vi "readAI.vi"(8 "error in (no error)":errorcluster, 10 "Samples To Read":i32=1000, 11 "DAQ Channel To Read":refnum<k21>) -> (0 "error out":errorcluster, 2 "Average":dbl, 3 "Samples":dbl[](array[numeric]) format="%0.2f")   [LabVIEW 2015]
uses:
  <vilib>/DAQmx/read.llb/DAQmx Read (Analog 1D DBL 1Chan NSamp).vi
  <vilib>/DAQmx/configure/timing.llb/DAQmx Timing (Sample Clock).vi
  <vilib>/DAQmx/miscellaneous.llb/DAQmx Fill In Error Info.vi
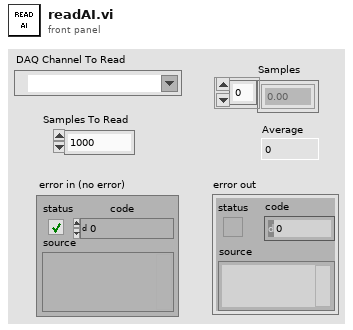
[diagram p1: front panel]
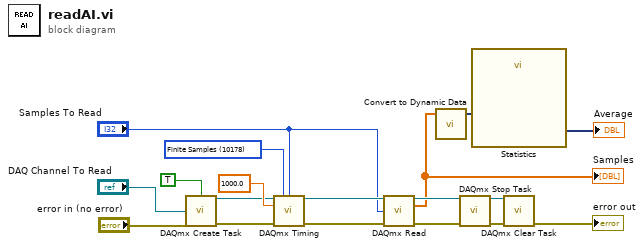
[diagram p0: block diagram]
diagram:
  w14 = 10178 items=["Finite Samples"=10178, "Continuous Samples"=10123, "Hardware Timed Single Point"=12522] ("sample mode")
  n1 = call <vilib>:"DAQmx Create Task.vi"("auto cleanup"=TRUE, "global virtual channels"="DAQ Channel To Read", "error in"="error in (no error)") -> ("task out"=w15:refnum<k21>, "error out"=w17:errorcluster)  [unwired: 11 in]
  n2 = call-poly <vilib>:"DAQmx Timing.vi"("task/channels in"=w15, "sample mode"=w14, "samples per channel"="Samples To Read", "rate"=1000.0, "error in"=w17) -> ("task out"=w12:refnum<k21>, "error out"=w13:errorcluster)  [unwired: 9 in]
  n3 = call-poly <vilib>:"DAQmx Read.vi"("task/channels in"=w12, "number of samples per channel"="Samples To Read", "error in"=w13) -> ("task out"=w11:refnum<k21>, "data"=w3:dbl[], "error out"=w10:errorcluster)  [unwired: 10 in]
  "Samples" <- w3
  n4 = call "Convert to Dynamic Data"("Array"=w3) -> ("Dynamic Data Type"=w2:dynamicdata)  [unwired: 3 in]
  n5 = call <vilib>:"DAQmx Stop Task.vi"("task/channels in"=w11, "error in"=w10) -> ("task out"=w9:refnum<k21>, "error out"=w8:errorcluster)  [unwired: 12 in]
  n6 = call "Statistics"("Signals"=w2) -> ("Arithmetic Mean"=→"Average":dynamicdata)  [unwired: 25 in, 1 out]
  n7 = call <vilib>:"DAQmx Clear Task.vi"("task in"=w9, "error in"=w8) -> ("error out"=→"error out":errorcluster)  [unwired: 13 in]
